vi "Read Analog.vi"(8 "error in (no error)":errorcluster, 10 "Pin":u8 max=7 step=1, 11 "VISA resource name":refnum<visa-resource-name>) -> (0 "error out":errorcluster, 2 "analog out":i32, 3 "VISA resource name out":refnum<visa-resource-name>)   [LabVIEW 2022 SP3, in "usbtmc_scpi_labtool.lvlib"]
uses:
  usbtmc_scpi_labtool.lvlib
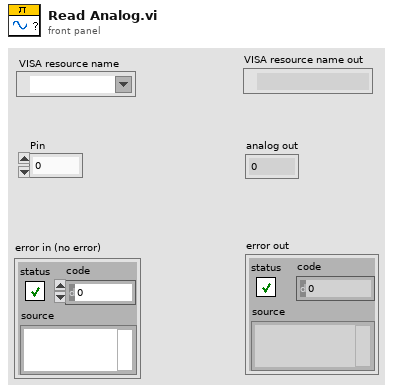
[diagram p1: front panel]
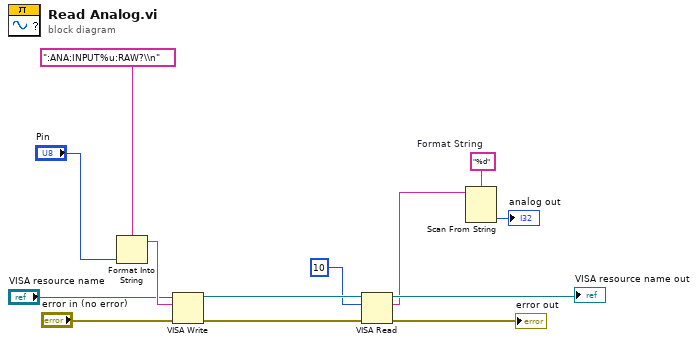
[diagram p0: block diagram]
diagram:
  w8 = "%d"  # Format String
  n1 = Format Into String(format string=":ANA:INPUT%u:RAW?\\n", "Pin") -> (resulting string=w12:string)  [unwired: 2 in, 1 out]
  n2 = VISA Write(VISA resource name="VISA resource name", write buffer=w12, error in (no error)="error in (no error)") -> (VISA resource name out=w3:refnum<visa-resource-name>, error out=w2:errorcluster)  [unwired: 1 out]
  n3 = VISA Read(VISA resource name=w3, byte count=u32 10, error in (no error)=w2) -> (VISA resource name out=→"VISA resource name out":refnum<visa-resource-name>, read buffer=w5:string, error out=→"error out":errorcluster)  [unwired: 1 out]
  n4 = Scan From String(format string=w8, input string=w5) -> (output 1=→"analog out":i32)  [unwired: 3 in, 3 out]
